vi "ToggleSingleOutput.vi"(1 "Boolean":bool=TRUE) -> (0 "Numeric":i32)   [LabVIEW 2013]
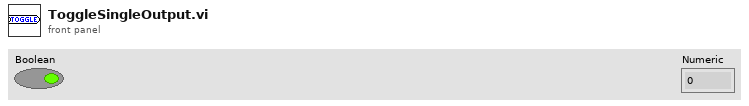
[diagram p1: front panel]
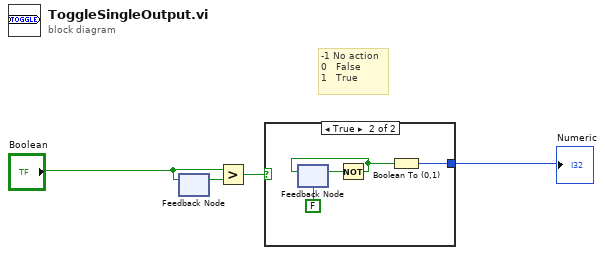
[diagram p0: block diagram]
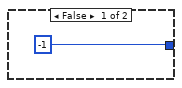
[diagram p2: hidden frame]
diagram:
  # "-1 No action\n0   False\n1   True"
  n1 = feedback #1() -> (w4:bool)  [unwired: 1 in]
  n2 = feedback-in #1("Boolean") -> ()
  n3 = Greater?(x="Boolean", y=w4) -> (0:w3:bool)
  n4 = case shown="True" w3 {
    tunnel: [-1 w7] -> w1
    frame False {
    }
    frame True {
      n5 = feedback #2(FALSE) -> (w8:bool)
      n6 = Not(x=w8) -> (.not. x?=w6:bool)
      n7 = feedback-in #2(w6) -> ()
      n8 = Boolean To (0,1)(Boolean=w6) -> (0, 1=w7:i16)
    }
  }
  "Numeric" <- w1
